vi "Grid Major Visible Write.vi"(8 "error in (no error)":errorcluster, 9 "Grid Major Visible?":bool, 11 "3D Plot.lvclass in":refnum<class "3D Plot.lvclass">) -> (0 "error out":errorcluster, 3 "3D Plot.lvclass out":refnum<class "3D Plot.lvclass">)   [LabVIEW 2020, in "3D Plot.lvclass"]
uses:
  3D Plot.lvclass
  3D Plot.lvclass/3D Plot.ctl
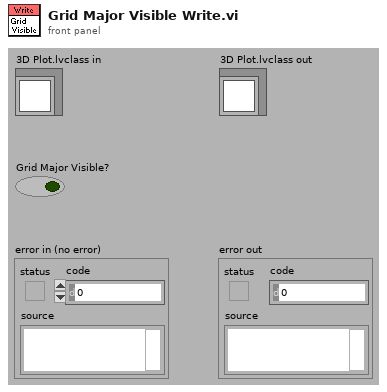
[diagram p1: front panel]
types:
  T1 = cluster{"Draw Major Grid X":bool, "Draw Major Grid Y":bool, "Draw Major Grid Z":bool}
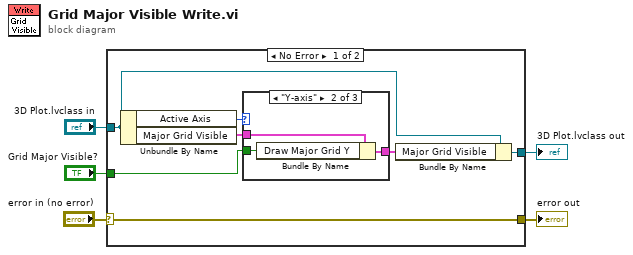
[diagram p0: block diagram]
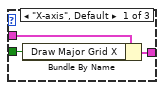
[diagram p2: hidden frame]
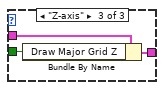
[diagram p3: hidden frame]
diagram:
  n1 = case shown="No Error" "error in (no error)" {
    selector: "error in (no error)" -> [w6 w22]
    tunnel: "Grid Major Visible?" -> [w12 _]
    tunnel: "3D Plot.lvclass in" -> [w8 w23]
    tunnel: [w7 w23] -> w3
    tunnel: [w6 w22] -> w1
    frame No Error {
      n2 = Unbundle By Name(w8) -> ("Active Axis"=w9:enum16{"X-axis", "Y-axis", "Z-axis"}, "Major Grid Visible"=w10:T1)
      n3 = case shown="\"Y-axis\"" w9 {
        tunnel: w10 -> [w15 w16 w20]
        tunnel: w12 -> [w14 w18 w21]
        tunnel: [w13 w17 w19] -> w11
        frame "X-axis", Default {
          n4 = Bundle By Name(cluster=w15, "Draw Major Grid X"=w14) -> (w13:T1)
        }
        frame "Y-axis" {
          n5 = Bundle By Name(cluster=w16, "Draw Major Grid Y"=w18) -> (w17:T1)
        }
        frame "Z-axis" {
          n6 = Bundle By Name(cluster=w20, "Draw Major Grid Z"=w21) -> (w19:T1)
        }
      }
      n7 = Bundle By Name(cluster=w8, "Major Grid Visible"=w11) -> (w7:refnum<class "3D Plot.lvclass">)
    }
    frame Error {
    }
  }
  "error out" <- w1
  "3D Plot.lvclass out" <- w3
